vi "load settings.vi"(8 "error in (no error)":errorcluster) -> (0 "error out":errorcluster, 3 "XML Elements":string[](array[string]))   [LabVIEW 2011]
uses:
  Controls/Full_90 Degree Pulse Settings.ctl
  Controls/90D_Delay Settings.ctl
  Controls/90D_Preliminary Settings.ctl
  Controls/90D_Pulse Settings.ctl
  Controls/Acquisition Settings.ctl
  Controls/Full_CPMG Degree Pulse Settings.ctl
  Controls/CPMG_Delay Settings.ctl
  Controls/CPMG_Preliminary Settings.ctl
  Controls/CPMG_Pulse Settings.ctl
  Controls/Full_T1 Degree Pulse Settings.ctl
  Controls/T1_Preliminary Settings.ctl
  Controls/T1_Pulse Settings.ctl
  Controls/T1_Delay Settings.ctl
  Controls/Hardware Control.ctl
  Functional Globals/Pulse Parameters.ctl
  Functional Globals/Hardware Parameters.ctl
  <vilib>/Utility/xml.llb/Read From XML File(array).vi
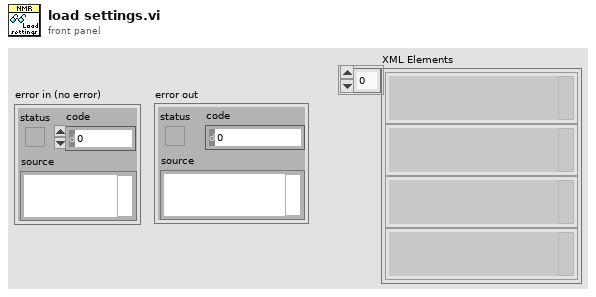
[diagram p1: front panel]
types:
  T1 = typedef "Hardware Parameters.ctl" = enum16{"Initialize", "Set Hardware Settings", "Get Hardware Settings", "Get Hardware CMD String"}
  T2 = typedef "Pulse Parameters.ctl" = enum16{"Initialize", "Set T1 Pulse Settings", "Set 90 Degree Pulse Settings", "Set CPMG Pulse Settings", "Get T1 Settings", "Get CPMG Settings", "Get 90 Degree Settings"}
  T3 = typedef "Hardware Control.ctl" = cluster{"Number Samples":u16, "Time Between Points":dbl, "Gain2 (dB)":i8, "CuttOff Freq1[MHz]":u8, "CuttOff Freq2[MHz]":u8, "Frequency":dbl, "Phase":u16, "Power Level":u16, "Send Pulse":bool, "Reset DDS":bool, "TX CTRL":bool, "RX CTRL":bool, "Gain1 (dB)":i8, "Set DDS":bool, "Start AQS":bool, "Units":u8}
  T4 = typedef "Full_T1 Degree Pulse Settings.ctl" = cluster{"Preliminary Settings":T5, "Pulse Settings":T6, "Acquisition Settings":T7, "Delay Settings":T8}
  T5 = typedef "T1_Preliminary Settings.ctl" = cluster{"Nº of Scans (ns)":u16, "Pulse Frequency":dbl, "Nº of Vd":u16}
  T6 = typedef "T1_Pulse Settings.ctl" = cluster{"Duration Signal P2":dbl, "Power Level P2":u16, "Phase P2":u16, "P2 Unit":u8, "Duration Signal P1":dbl, "Power Level P1":u16, "Phase P1":u16, "P1 Unit":u8}
  T7 = typedef "Acquisition Settings.ctl" = cluster{"Number Samples":u16, "Time Between Points":dbl, "Unit":u8}
  T8 = typedef "T1_Delay Settings.ctl" = cluster{"Delay d1":dbl, "Delay d2":dbl, "d1 Unit":u8, "d2 Unit":u8, "Delay d30":dbl, "d30 Unit":u8, "Vd Unit":u8, "Vd Values":string}
  T9 = typedef "Full_CPMG Degree Pulse Settings.ctl" = cluster{"Acquisition Settings":T7, "Delay Settings":T10, "Preliminary Settings":T11, "Pulse Settings":T12}
  T10 = typedef "CPMG_Delay Settings.ctl" = cluster{"Delay d1":dbl, "Delay d2":dbl, "d1 Unit":u8, "d2 Unit":u8, "Delay d3":dbl, "d3 Unit":u8, "Delay d4":dbl, "d4 Unit":u8}
  T11 = typedef "CPMG_Preliminary Settings.ctl" = cluster{"Nº of Scans (ns)":u16, "Pulse Frequency":dbl, "Nº of Echoes (ne)":u16}
  T12 = typedef "CPMG_Pulse Settings.ctl" = cluster{"Duration Signal P1":dbl, "Power Level P1":u16, "Phase P1":u16, "P1 Unit":u8, "Duration Signal P2":dbl, "Power Level P2":u16, "Phase P2":u16, "P2 Unit":u8}
  T13 = typedef "Full_90 Degree Pulse Settings.ctl" = cluster{"Delay Settings":T14, "Preliminary Settings":T15, "Pulse Settings":T16, "Acquisition Settings":T7}
  T14 = typedef "90D_Delay Settings.ctl" = cluster{"Delay d1":dbl, "Delay d2":dbl, "d1 Unit":u8, "d2 Unit":u8}
  T15 = typedef "90D_Preliminary Settings.ctl" = cluster{"Nº of Scans (ns)":u16, "Pulse Frequency":dbl}
  T16 = typedef "90D_Pulse Settings.ctl" = cluster{"Duration Signal P1":dbl, "Power Level":u16, "Phase":u16, "P1 Units":u8}
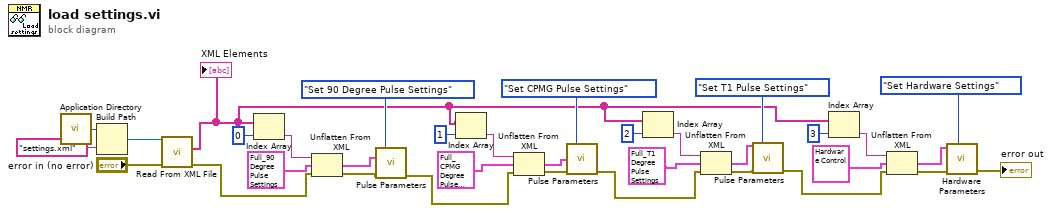
[diagram p0: block diagram]
diagram:
  n1 = call <vilib>:"Application Directory.vi"() -> ("Application Directory"=w16:path)
  n2 = Build Path(base path=w16, name or relative path="settings.xml") -> (appended path=w15:path)
  n3 = call-poly <vilib>:"Read From XML File.vi"("error in (no error)"="error in (no error)", "XML File Path"=w15) -> ("error out"=w25:errorcluster, "XML Elements"=w11:string[])  [unwired: 7 in, 1 out]
  "XML Elements" <- w11
  n4 = Index Array(array=w11, index=0) -> (element=w23:string)
  n5 = Unflatten From XML(xml string=w23, type=T13 {"Delay Settings"={"Delay d1"=10.0, "Delay d2"=0.0, "d1 Unit"=0, "d2 Unit"=0}, "Preliminary Settings"={"Nº of Scans (ns)"=3, "Pulse Frequency"=10000000.0}, "Pulse Settings"={"Duration Signal P1"=20.0, "Power Level"=1023, "Phase"=90, "P1 Units"=0}, "Acquisition Settings"={"Number Samples"=2000, "Time Between Points"=0.0, "Unit"=0}} ("90 Degree Pulse Sequence"), error in (no error)=w25) -> (value=w13:T13, error out=w12:errorcluster)
  n6 = call "Pulse Parameters.vi"("action"=Pulse_Parameters."Set 90 Degree Pulse Settings", "90 Degree Pulse Sequence"=w13, "error in"=w12) -> ("error out"=w10:errorcluster)  [unwired: 5 in, 7 out]
  n7 = Index Array(array=w11, index=1) -> (element=w26:string)
  n8 = Unflatten From XML(xml string=w26, type=T9 {"Acquisition Settings"={"Number Samples"=2000, "Time Between Points"=0.0, "Unit"=0}, "Delay Settings"={"Delay d1"=10.0, "Delay d2"=0.0, "d1 Unit"=0, "d2 Unit"=0, "Delay d3"=0.0, "d3 Unit"=0, "Delay d4"=0.0, "d4 Unit"=0}, "Preliminary Settings"={"Nº of Scans (ns)"=3, "Pulse Frequency"=10000000.0, "Nº of Echoes (ne)"=3}, "Pulse Settings"={"Duration Signal P1"=20.0, "Power Level P1"=1023, "Phase P1"=90, "P1 Unit"=0, "Duration Signal P2"=20.0, "Power Level P2"=1023, "Phase P2"=90, "P2 Unit"=0}} ("CPMG Pulse Sequence"), error in (no error)=w10) -> (value=w8:T9, error out=w9:errorcluster)
  n9 = call "Pulse Parameters.vi"("action"=Pulse_Parameters."Set CPMG Pulse Settings", "CPMG Pulse Sequence"=w8, "error in"=w9) -> ("error out"=w7:errorcluster)  [unwired: 5 in, 7 out]
  n10 = Index Array(array=w11, index=2) -> (element=w29:string)
  n11 = Unflatten From XML(xml string=w29, type=T4 {"Preliminary Settings"={"Nº of Scans (ns)"=3, "Pulse Frequency"=10000000.0, "Nº of Vd"=3}, "Pulse Settings"={"Duration Signal P2"=20.0, "Power Level P2"=1023, "Phase P2"=90, "P2 Unit"=0, "Duration Signal P1"=20.0, "Power Level P1"=1023, "Phase P1"=90, "P1 Unit"=0}, "Acquisition Settings"={"Number Samples"=2000, "Time Between Points"=0.0, "Unit"=0}, "Delay Settings"={"Delay d1"=10.0, "Delay d2"=0.0, "d1 Unit"=0, "d2 Unit"=0, "Delay d30"=0.0, "d30 Unit"=0, "Vd Unit"=0, "Vd Values"="0"}} ("T1 Pulse Sequence"), error in (no error)=w7) -> (value=w6:T4, error out=w5:errorcluster)
  n12 = call "Pulse Parameters.vi"("T1 Pulse Sequence"=w6, "action"=Pulse_Parameters."Set T1 Pulse Settings", "error in"=w5) -> ("error out"=w4:errorcluster)  [unwired: 5 in, 7 out]
  n13 = Index Array(array=w11, index=3) -> (element=w32:string)
  n14 = Unflatten From XML(xml string=w32, type=T3 {"Number Samples"=5000, "Time Between Points"=0.0, "Gain2 (dB)"=20, "CuttOff Freq1[MHz]"=9, "CuttOff Freq2[MHz]"=1, "Frequency"=8000000.0, "Phase"=180, "Power Level"=512, "Send Pulse"=FALSE, "Reset DDS"=FALSE, "TX CTRL"=FALSE, "RX CTRL"=FALSE, "Gain1 (dB)"=15, "Set DDS"=FALSE, "Start AQS"=FALSE, "Units"=0} ("Cluster"), error in (no error)=w4) -> (value=w3:T3, error out=w2:errorcluster)
  n15 = call "Hardware Parameters.vi"("action"=Hardware_Parameters."Set Hardware Settings", "error in"=w2, "Hardware Parameters"=w3) -> ("error out"=→"error out":errorcluster)  [unwired: 7 in, 1 out]
